vi "getProtocolMode.vi"(8 "error in (no error)":errorcluster, 11 "pHandle":u32) -> (0 "error out":errorcluster, 2 "return type":i32, 3 "pBaudRate":u32)   [LabVIEW 2011, in "sbgLabView.lvlib"]
uses:
  sbgLabView.lvlib
  sbgMatLab.dll
panel:
  out "pUartOptionsStr":string
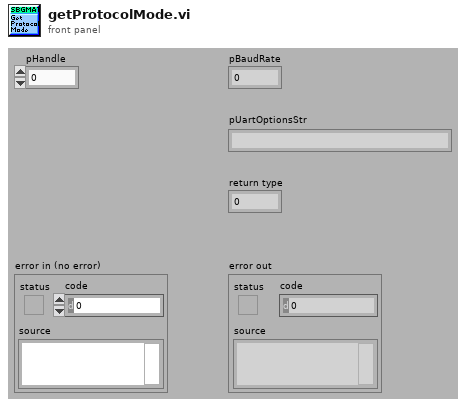
[diagram p1: front panel]
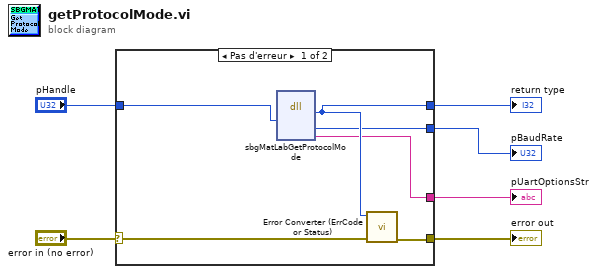
[diagram p0: block diagram]
diagram:
  n1 = case shown="Pas d'erreur" "error in (no error)" {
    selector: "error in (no error)" -> [w9 w13]
    tunnel: [w8 w13] -> w5
    tunnel: [w12 _] -> w4
    tunnel: "pHandle" -> [w11 _]
    tunnel: [w10 _] -> w2
    tunnel: [w7 _] -> w1
    frame No Error {
      n2 = dll-call lib="C:/SBG-Systems/remote/projects/software/projects/labviewExample/sbgLabView/sbgMatLab.*" fn="sbgMatLabGetProtocolMode"("pHandle"=w11) -> ("return type"=w12:i32, "pBaudRate"=w10:u32, "uartOptionsStr"=w7:string)  [unwired: 6 in, 2 out]
      n3 = call "Error Converter (ErrCode or Status).vi"("error in (no error)"=w9, "error code"=w12) -> ("error out"=w8:errorcluster)  [unwired: 9 in]
    }
    frame Error {
    }
  }
  "return type" <- w4
  "pBaudRate" <- w2
  "error out" <- w5
  "pUartOptionsStr" <- w1
